vi "Match Pattern in Column Name Array.vi"(3 "Match Pattern Regex":string[](array[string]), 4 "Column Name Array":string[](array[string]), 5 "Not Found Name":string) -> (0 "Regex Index":i32, 1 "Column Index":i32, 2 "Matching Name":string)   [LabVIEW 2020, in "Old Basic Fields.lvlib"]
uses:
  Old Basic Fields.lvlib
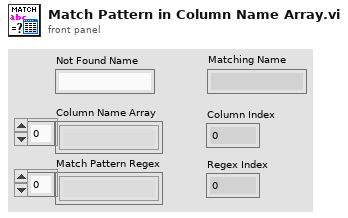
[diagram p1: front panel]
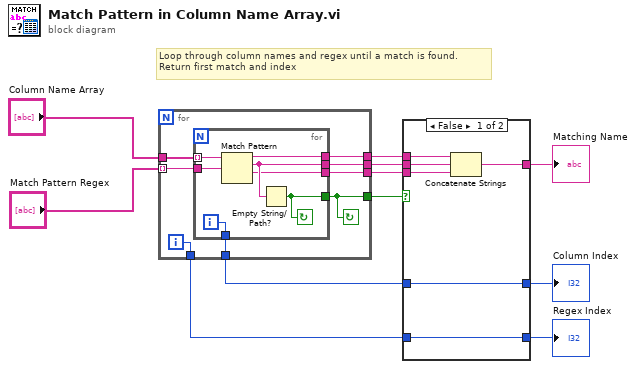
[diagram p0: block diagram]
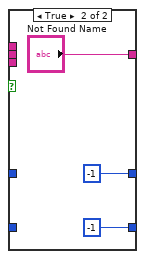
[diagram p2: hidden frame]
diagram:
  # "Loop through column names and regex until a match is found.\nReturn first match and index"
  n1 = for {
    tunnel: "Match Pattern Regex" -> [w18] mode=indexing
    tunnel: "Column Name Array" -> [w19]
    tunnel: [w17] -> w3
    tunnel: [w16] -> w2
    tunnel: [w15] -> w1
    tunnel: [w14] -> w11
    tunnel: [w13] -> w7
    tunnel: [w12] -> w6
    i -> [w13]
    stop <- w14 continue-if-true
    n2 = for {
      tunnel: w19 -> [w26] mode=indexing
      tunnel: w18 -> [w25]
      tunnel: [w24] -> w14
      tunnel: [w23] -> w17
      tunnel: [w22] -> w16
      tunnel: [w21] -> w15
      tunnel: [w20] -> w12
      i -> [w20]
      stop <- w24 continue-if-true
      n3 = Match Pattern(string=w26, regular expression=w25) -> (before substring=w23:string, match substring=w22:string, after substring=w21:string)  [unwired: 1 in, 1 out]
      n4 = Empty String/Path?(string/path=w22) -> (empty?=w24:bool)
    }
  }
  n5 = case shown="False" w11 {
    tunnel: [w27 "Not Found Name"] -> w8
    tunnel: w7 -> [w31 _]
    tunnel: w6 -> [w32 _]
    tunnel: [w32 -1] -> w5
    tunnel: [w31 -1] -> w4
    tunnel: w3 -> [w30 _]
    tunnel: w2 -> [w29 _]
    tunnel: w1 -> [w28 _]
    frame False {
      n6 = Concatenate Strings(w30, w29, w28) -> (w27:string)
    }
    frame True {
    }
  }
  "Matching Name" <- w8
  "Column Index" <- w5
  "Regex Index" <- w4
